vi "format AI settings.vi"(10 "Analoge In Settings":T1) -> (3 "analogue in settings (for type) out":T2)   [LabVIEW 2018]
panel:
  in  "analogue in settings (for type) in":T2
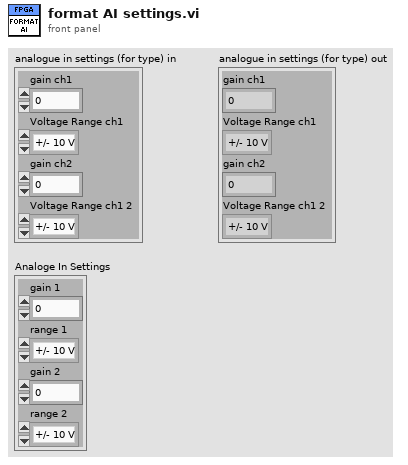
[diagram p1: front panel]
types:
  T1 = cluster{"gain 1":dbl, "range 1":enum16{"+/- 10 V", "+/- 5 V", "+/- 2 V", "+/- 1 V"}, "gain 2":dbl, "range 2":enum16{"+/- 10 V", "+/- 5 V", "+/- 2 V", "+/- 1 V"}}
  T2 = cluster{"gain ch1":fxp<+,18,6>, "Voltage Range ch1":enum8{"+/- 10 V", "+/- 5 V", "+/- 2 V", "+/- 1 V"}, "gain ch2":fxp<+,18,6>, "Voltage Range ch1 2":enum8{"+/- 10 V", "+/- 5 V", "+/- 2 V", "+/- 1 V"}}
  T3 = enum16{"+/- 10 V", "+/- 5 V", "+/- 2 V", "+/- 1 V"}
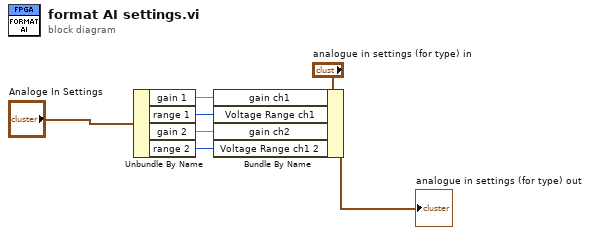
[diagram p0: block diagram]
diagram:
  n1 = Unbundle By Name("Analoge In Settings") -> ("gain 1"=w3:dbl, "range 1"=w4:T3, "gain 2"=w5:dbl, "range 2"=w6:T3)
  n2 = Bundle By Name(cluster="analogue in settings (for type) in", "gain ch1"=w3, "Voltage Range ch1"=w4, "gain ch2"=w5, "Voltage Range ch1 2"=w6) -> (→"analogue in settings (for type) out":T2)
